vi "IMAQdx_get_ROI.vi"(10 "Session In":T1) -> (2 "ROI":u32[](array[numeric]), 3 "Session Out":T1)   [LabVIEW 2019]
doc: "Use a property node to find the current ROI of the camera."
uses:
  <vilib>/userDefined/High Color/IMAQdx.ctl
  <resource>/objmgr/imaqdx.rc
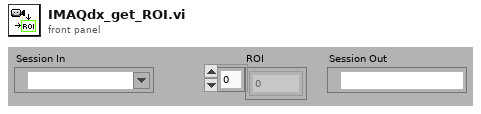
[diagram p1: front panel]
types:
  T1 = typedef "IMAQdx.ctl" = refnum<k21>
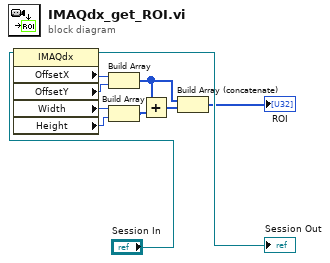
[diagram p0: block diagram]
diagram:
  n1 = property class="IMAQdx"(reference="Session In") -> (reference out=→"Session Out":T1, "OffsetX"=w2:u32, "OffsetY"=w1:u32, "Width"=w3:u32, "Height"=w4:u32)  [unwired: 1 in, 1 out]
  n2 = Build Array(w2, w1) -> (w7:u32[])
  n3 = Build Array(w3, w4) -> (w5:u32[])
  n4 = Add(x=w7, y=w5) -> (x+y=w6:u32[])
  n5 = Build Array (concatenate)(w7, w6) -> (→"ROI":u32[])
